vi "set_claster_value_from_eDoc_by_name.vi"(5 "little-endian arrays (T)":bool=TRUE, 8 "error in (no error)":errorcluster, 10 "arrayOfElements":T1[](array[typedef]), 11 "dataType in":variant) -> (0 "error out":errorcluster, 3 "Data dup":variant)   [LabVIEW 2015, in "BSON_convertors_Library.lvlib"]
doc: "Created by Artem Shevelev\nLabVIEW Portal profile: http://www.labviewportal.org/memberlist.php?mode=viewprofile&u=2340\ne-mail: artem.sh@gmail.com\nshevelev.pro"
uses:
  BSON_convertors_Library.lvlib
  typedefs/BSONelement.ctl
  typedefs/dataType.ctl
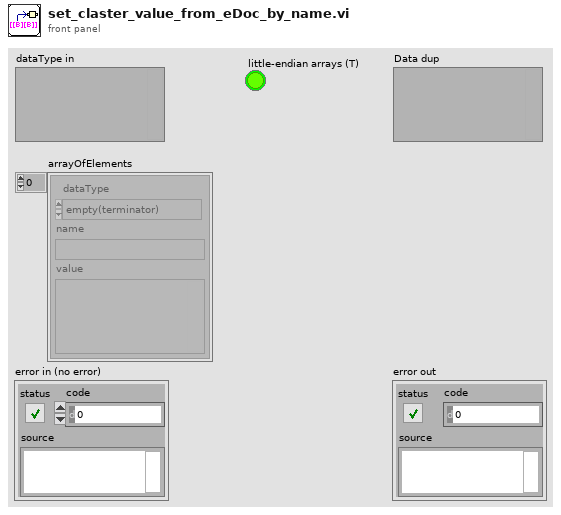
[diagram p1: front panel]
types:
  T1 = typedef "BSON_convertors_Library.lvlib/BSONelement.ctl" = cluster{"dataType":T2, "name":string, "value":variant}
  T2 = typedef "BSON_convertors_Library.lvlib/dataType.ctl" = enum8{"empty(terminator)", "double", "string", "document", "array", "binary", "Deprecated(Undefined)", "ObjectId", "boolean", "UTC datetime", "Null value", "cstring", "Deprecated(DBPointer)", "JavaScript", "Deprecated(Symbol)", "code_w_s", "int32", "uint64", "int64", "ext (decimal128)", "Min key", "Max key"}
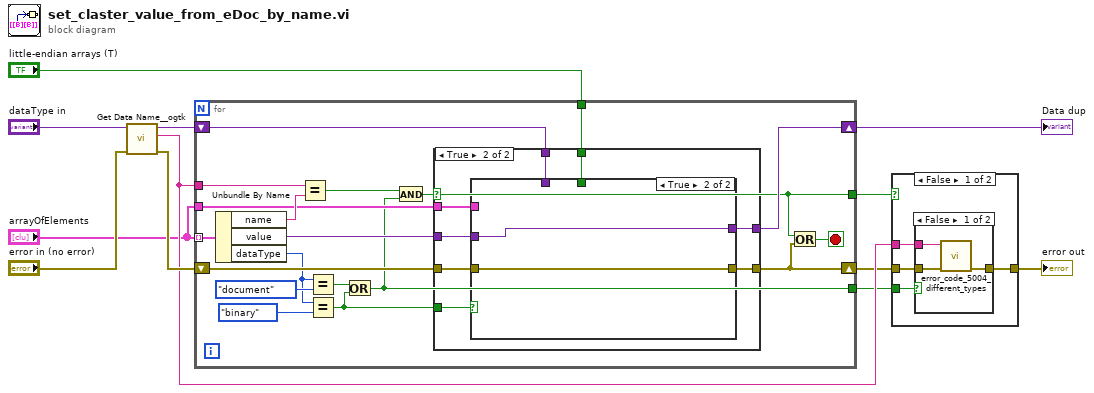
[diagram p0: block diagram]
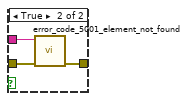
[diagram p2: hidden frame]
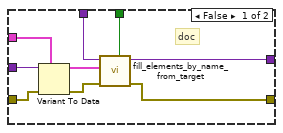
[diagram p5: hidden frame]
diagram:
  n1 = call <userlib>:"Get Data Name__ogtk.vi"("error in (no error)"="error in (no error)", "Data"="dataType in") -> ("error out"=w12:errorcluster, "Data Name"=w10:string, "Data dup"=w9:variant)  [unwired: 7 in]
  n2 = for {
    tunnel: "arrayOfElements" -> [w31] mode=indexing
    tunnel: w10 -> [w30]
    tunnel: [w20] -> w7
    shift-right: [w23] -> w6
    shift-left: w12 -> [w25]
    shift-right: [w26] -> w5
    shift-left: w9 -> [w27]
    tunnel: [w15] -> w3
    tunnel: "arrayOfElements" -> [w19]
    tunnel: "little-endian arrays (T)" -> [w13]
    stop <- w24 stop-if-true
    n3 = Unbundle By Name(w31) -> ("name"=w29:string, "value"=w28:variant, "dataType"=w18:T2)
    n4 = Equal?(x=w30, y=w29) -> (x = y?=w21:bool)
    n5 = Equal?(x=w18, y=dataType."document") -> (x = y?=w16:bool)
    n6 = Equal?(x=w18, y=dataType."binary") -> (x = y?=w14:bool)
    n7 = Or(x=w16, y=w14) -> (x .or. y?=w15:bool)
    n8 = And(x=w21, y=w15) -> (x .and. y?=w20:bool)
    n9 = case shown="True" w20 {
      tunnel: w28 -> [_ w41]
      tunnel: w27 -> [w33 w37]
      tunnel: [w33 w36] -> w26
      tunnel: w25 -> [w32 w40]
      tunnel: [w32 w38] -> w23
      tunnel: w19 -> [_ w39]
      tunnel: w14 -> [_ w35]
      tunnel: w13 -> [_ w34]
      frame False {
      }
      frame True {
        n10 = case shown="True" w35 {
          tunnel: w41 -> [w50 w52]
          tunnel: w40 -> [w49 w51]
          tunnel: w39 -> [w48 _]
          tunnel: [w45 w51] -> w38
          tunnel: w37 -> [w44 _]
          tunnel: [w43 w52] -> w36
          tunnel: w34 -> [w42 _]
          frame False {
            # "doc"
            n11 = Variant To Data(error in=w49, type=w48, Variant=w50) -> (data=w47:T1[], error out=w46:errorcluster)
            n12 = call "fill_elements_by_name_from_target.vi"("little-endian arrays (T)"=w42, "error in (no error)"=w46, "arrayOfElements"=w47, "dataType in"=w44) -> ("error out"=w45:errorcluster, "dataType out"=w43:variant)  [unwired: 6 in]
          }
          frame True {
          }
        }
      }
    }
    n13 = Or(x=w20, y=w23) -> (x .or. y?=w24:bool)
  }
  "Data dup" <- w5
  n14 = case shown="False" w7 {
    tunnel: w6 -> [w56 w63]
    tunnel: w10 -> [w55 _]
    tunnel: [w54 w63] -> w8
    tunnel: w3 -> [w53 _]
    frame False {
      n15 = case shown="False" w53 {
        tunnel: w56 -> [w59 w62]
        tunnel: w55 -> [w57 w61]
        tunnel: [w58 w60] -> w54
        frame False {
          n16 = call "error_code_5004_different_types.vi"("error in (no error)"=w59, "name"=w57) -> ("error out"=w58:errorcluster)  [unwired: 9 in]
        }
        frame True {
          n17 = call "error_code_5001_element_not_found.vi"("error in (no error)"=w62, "name"=w61) -> ("error out"=w60:errorcluster)  [unwired: 9 in]
        }
      }
    }
    frame True {
    }
  }
  "error out" <- w8
